vi "Simple FPGA Add.vi"(9 "y":i32, 10 "x":i32) -> (2 "x+y":i32)   [LabVIEW 2018]
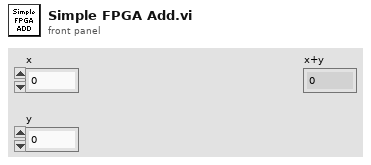
[diagram p1: front panel]
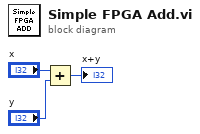
[diagram p0: block diagram]
diagram:
  n1 = Add(x="x", y="y") -> (x+y=→"x+y":i32)
